vi "struct_ads_T_pw.vi"(8 "Error (Input)":errorcluster, 9 "Loading in kg/kg (Input)":dbl, 10 "Pressure in Pa (Input)":dbl, 11 "Reference working pair (Input)":i64) -> (0 "Error (Output)":errorcluster caption="Error(Output)", 3 "Temperature in K (Output)":dbl)   [LabVIEW 2017]
doc: "ads_T_pw:\n * ---------\n *\n * Calculates equilibrium temperature in K depending on equilibrium pressure p\n * in Pa and equilibrium loading w in kg/kg.\n *\n * Parameters:\n * -----------\n * double p_Pa:\n * Equilibrium pressure in Pa.\n * double w_kgkg:\n * Equilibrium loading in kg/kg.\n * struct *WorkingPair:\n * Pointer of WorkingPair-struct.\n *\n * Returns:\n * --------\n * double:\n * Equilibrium temperature in K.\n *\n * Remarks:\n * --------\n * Function uses equation of states implemented for calculation of vapor\n * pressure, saturated liquid density, derivative of vapor pressure wrt.\n * temperature, and derivative of saturated liquid density wrt. temperature\n * when isotherm of working pair is based on volumetric approach (e.g.\n * Dubinin theory).\n *\n * History:\n * --------\n * 07/13/2021, by Jannik Driesel (supervised by Mirko Engelpracht):\n * First implementation."
uses:
  data/win32bit/libsorpPropLib.dll
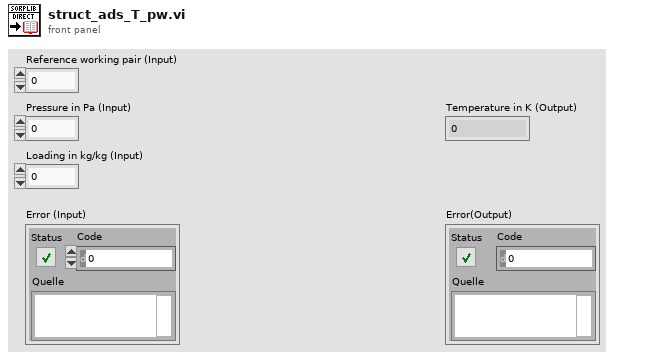
[diagram p1: front panel]
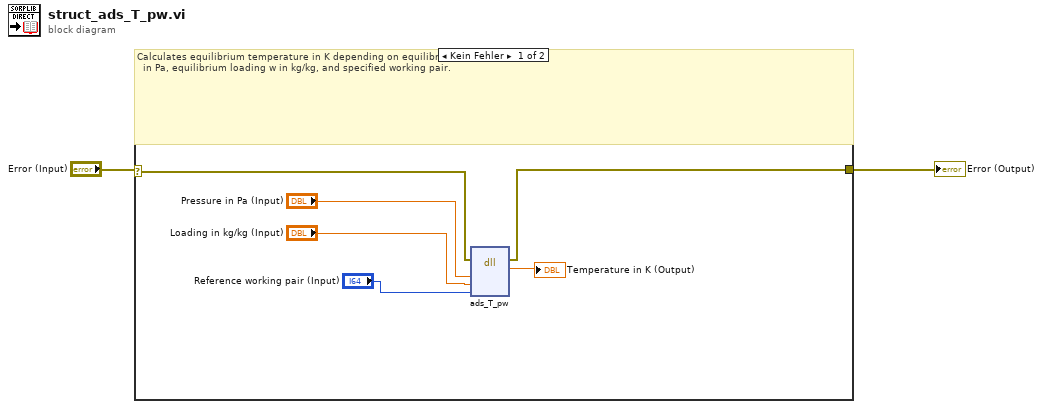
[diagram p0: block diagram]
diagram:
  n1 = case shown="Kein Fehler" "Error (Input)" {
    selector: "Error (Input)" -> [w6 w9]
    tunnel: [w5 w9] -> w1
    frame No Error {
      # "Calculates equilibrium temperature in K depending on equilibrium pressure p\n  in Pa, equilibrium loading w in kg/kg, and specified working pair."
      n2 = dll-call lib="D:/Driesel/SorpLibLocal/LabVIEW_wrapper/data/win32bit/libsorpPropLib.dll" fn="ads_T_pw"(error in=w6, "p_Pa"="Pressure in Pa (Input)", "w_kgkg"="Loading in kg/kg (Input)", "workingPair"="Reference working pair (Input)") -> (error out=w5:errorcluster, "T_K"=→"Temperature in K (Output)":dbl)  [unwired: 5 in, 1 out]
    }
    frame Error {
      # "Error - No calculations"
    }
  }
  "Error (Output)" <- w1
